vi "Destroy.vi"(0 "reference in":refnum<class "MusicPlayer.lvclass">, 11 "Error In":errorcluster) -> (4 "reference out":refnum<class "MusicPlayer.lvclass">, 15 "Error Out":errorcluster)   [LabVIEW 2022 SP3, in "MusicPlayer.lvclass"]
uses:
  MusicPlayer.lvclass
  MusicPlayer.lvclass/MusicPlayer.ctl
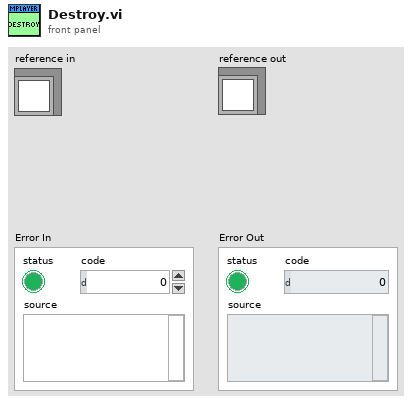
[diagram p1: front panel]
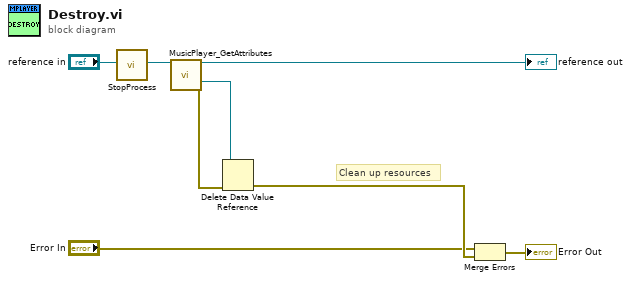
[diagram p0: block diagram]
diagram:
  # "Clean up resources"
  n1 = call "StopProcess.vi"("reference in"="reference in") -> ("reference out"=w1:refnum<class "MusicPlayer.lvclass">)  [unwired: 17 in, 1 out]
  n2 = call "MusicPlayer_GetAttributes.vi"("reference in"=w1) -> ("reference out"=→"reference out":refnum<class "MusicPlayer.lvclass">, "DataRef"=w5:refnum<data-value>, "error out"=w6:errorcluster)  [unwired: 11 in, 1 out]
  n3 = Delete Data Value Reference(data value reference=w5, error in=w6) -> (error out=w4:errorcluster)  [unwired: 1 out]
  n4 = Merge Errors("Error In", w4) -> (→"Error Out":errorcluster)
